vi "Append Warnign (SubVI).vi"(6 "Código W":i16, 7 "Descripcion":string, 9 "time stamp":timestamp) -> ()   [LabVIEW 2021, in "Control Vis.lvlib"]
uses:
  Control Vis.lvlib
panel:
  out "output array":T1(array[cluster])
  in  "Array in":T1(array[cluster])
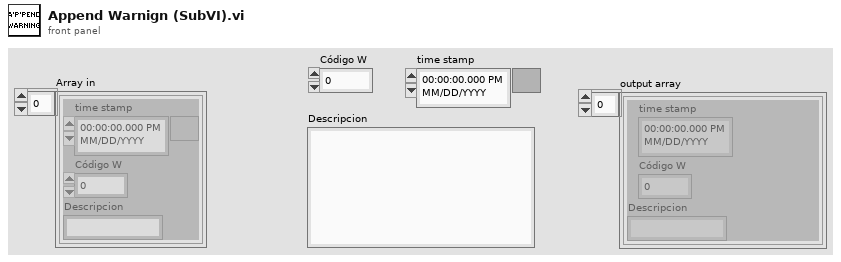
[diagram p1: front panel]
types:
  T1 = cluster{"time stamp":timestamp, "Código W":i16, "Descripcion":string}[]
  T2 = cluster{"time stamp":timestamp, "Código W":i16, "Descripcion":string}
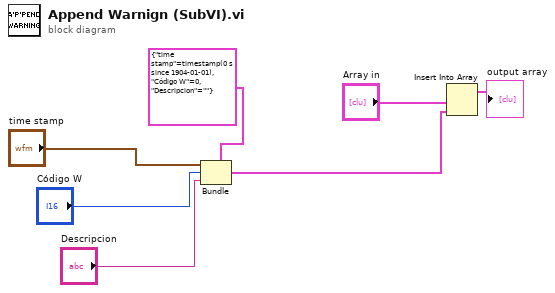
[diagram p0: block diagram]
diagram:
  n1 = Bundle(cluster=T2 {"time stamp"=timestamp(0 s since 1904-01-01), "Código W"=0, "Descripcion"=""} ("Warning"), "time stamp"="time stamp", "Código W"="Código W", "Descripcion"="Descripcion") -> (w5:T2)
  n2 = Insert Into Array(array="Array in", new element=w5) -> (→"output array":T1)  [unwired: 1 in]
